vi "GetDVRref.vi"(8 "error in (no error)":errorcluster, 10 "data value reference":refnum<data-value>, 11 "Arithmetic in":refnum<class "Arithmetic.lvclass">) -> (0 "error out":errorcluster, 1 "Arithmetic out":refnum<class "Arithmetic.lvclass">, 2 "data value reference":refnum<data-value>, 3 "Arithmetic out":refnum<class "Arithmetic.lvclass">)   [LabVIEW 2023, in "Arithmetic.lvclass"]
uses:
  Arithmetic.lvclass
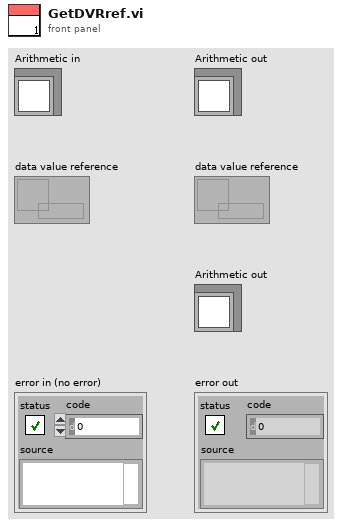
[diagram p1: front panel]
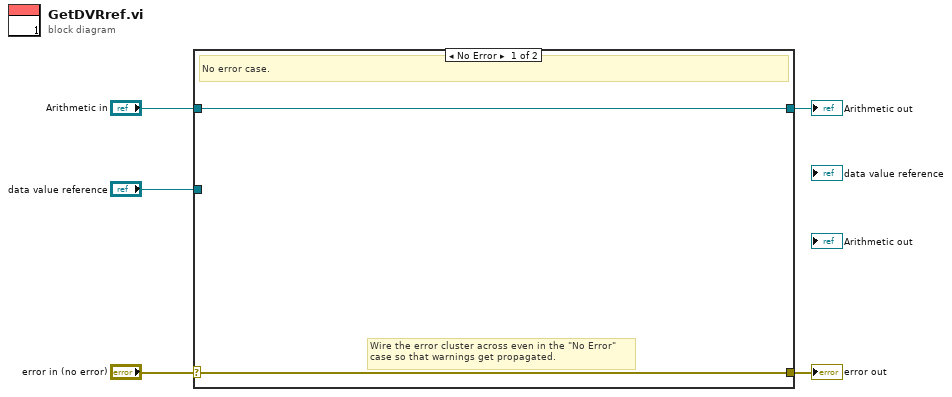
[diagram p0: block diagram]
diagram:
  n1 = case shown="No Error" "error in (no error)" {
    selector: "error in (no error)" -> [w7 w9]
    tunnel: [w7 w9] -> w4
    tunnel: [w6 w8] -> w2
    tunnel: "Arithmetic in" -> [w6 w8]
    tunnel: "data value reference" -> [_ _]
    frame No Error {
      # "Wire the error cluster across even in the \"No Error\"\ncase so that warnings get propagated."
      # "No error case."
    }
    frame Error {
      # "Error case."
    }
  }
  "error out" <- w4
  "Arithmetic out" <- w2
